vi "Initialization_default.vi"(8 "error in (no error)":errorcluster, 11 "Device Item Ref in":T3 format="%.0x") -> (0 "error out":errorcluster, 3 "Device Item Ref out":T3 format="%.0x")   [LabVIEW 2017, in "ALMA_10201-10401_O2SensorSim System Explorer.lvlib"]
uses:
  ALMA_10201-10401_O2SensorSim System Explorer.lvlib
  <vilib>/NI Veristand/Custom Device API/Custom Device Item Ref.ctl
  Engine/Par.ctl
  Engine/LambdaType.ctl
  <vilib>/NI Veristand/Custom Device API/Set Item Property (String).vi
  <vilib>/NI Veristand/Custom Device API/Custom Device API.lvlib
panel:
  in  "par":T1={"Loop time"={"Period [ms]"=0, "Processor"=0}, "COM"={"COM IP"="0.0.0.0", "COM port"=1, "Local port"=0, "Next_IP 1"=0, "Next_IP 2"=0, "Next_IP 3"=0, "Next_IP 4"=0}, "O2Sensor1"={"Lambda"={"LSU4.2 Lambda"=[], "LSU4.2 Ip"=[], "LSU4.9 Lambda"=[], "LSU4.9 Ip"=[], "LZA03 Lambda"=[], "LZA03 Ip"=[], "LZA08 Lambda"=[], "LZA08 Ip"=[], "Custom Lambda"=[], "Custom Ip"=[]}, "Temp"={"LSU4.2 Temp"=[], "LSU4.2 Ohm"=[], "LSU4.9 Temp"=[], "LSU4.9 Ohm"=[], "LZA03 Temp"=[], "LZA03 Ohm"=[], "LZA08 Temp"=[], "LZA08 Ohm"=[], "Custom Temp"=[], "Custom Ohm"=[]}, "Lambda Type"=0, "PID"={"Ki"=0.0, "Kp"=0.0, "Kd"=0.0, "FeedFW"=0.0}}, "O2Sensor2"={"Lambda"={"LSU4.2 Lambda"=[], "LSU4.2 Ip"=[], "LSU4.9 Lambda"=[], "LSU4.9 Ip"=[], "LZA03 Lambda"=[], "LZA03 Ip"=[], "LZA08 Lambda"=[], "LZA08 Ip"=[], "Custom Lambda"=[], "Custom Ip"=[]}, "Temp"={"LSU4.2 Temp"=[], "LSU4.2 Ohm"=[], "LSU4.9 Temp"=[], "LSU4.9 Ohm"=[], "LZA03 Temp"=[], "LZA03 Ohm"=[], "LZA08 Temp"=[], "LZA08 Ohm"=[], "Custom Temp"=[], "Custom Ohm"=[]}, "Lambda Type"=0, "PID"={"Ki"=0.0, "Kp"=0.0, "Kd"=0.0, "FeedFW"=0.0}}, "O2Sensor3"={"Lambda"={"LSU4.2 Lambda"=[], "LSU4.2 Ip"=[], "LSU4.9 Lambda"=[], "LSU4.9 Ip"=[], "LZA03 Lambda"=[], "LZA03 Ip"=[], "LZA08 Lambda"=[], "LZA08 Ip"=[], "Custom Lambda"=[], "Custom Ip"=[]}, "Temp"={"LSU4.2 Temp"=[], "LSU4.2 Ohm"=[], "LSU4.9 Temp"=[], "LSU4.9 Ohm"=[], "LZA03 Temp"=[], "LZA03 Ohm"=[], "LZA08 Temp"=[], "LZA08 Ohm"=[], "Custom Temp"=[], "Custom Ohm"=[]}, "Lambda Type"=0, "PID"={"Ki"=0.0, "Kp"=0.0, "Kd"=0.0, "FeedFW"=0.0}}, "O2Sensor4"={"Lambda"={"LSU4.2 Lambda"=[], "LSU4.2 Ip"=[], "LSU4.9 Lambda"=[], "LSU4.9 Ip"=[], "LZA03 Lambda"=[], "LZA03 Ip"=[], "LZA08 Lambda"=[], "LZA08 Ip"=[], "Custom Lambda"=[], "Custom Ip"=[]}, "Temp"={"LSU4.2 Temp"=[], "LSU4.2 Ohm"=[], "LSU4.9 Temp"=[], "LSU4.9 Ohm"=[], "LZA03 Temp"=[], "LZA03 Ohm"=[], "LZA08 Temp"=[], "LZA08 Ohm"=[], "Custom Temp"=[], "Custom Ohm"=[]}, "Lambda Type"=0, "PID"={"Ki"=0.0, "Kp"=0.0, "Kd"=0.0, "FeedFW"=0.0}}, "Board"=1, "Mode"=enum."SLSC Mode", "vendor.Num"=4141, "product.Num"=0} {"Board" items=["ALMA-10201", "ALMA-10401"]; "O2Sensor4"."Lambda Type" items=["LSU4.2", "LSU4.9", "LZA03", "LZA08", "Custom", "[mA]"]; "O2Sensor3"."Lambda Type" items=["LSU4.2", "LSU4.9", "LZA03", "LZA08", "Custom", "[mA]"]; "O2Sensor2"."Lambda Type" items=["LSU4.2", "LSU4.9", "LZA03", "LZA08", "Custom", "[mA]"]; "O2Sensor1"."Lambda Type" items=["LSU4.2", "LSU4.9", "LZA03", "LZA08", "Custom", "[mA]"]}
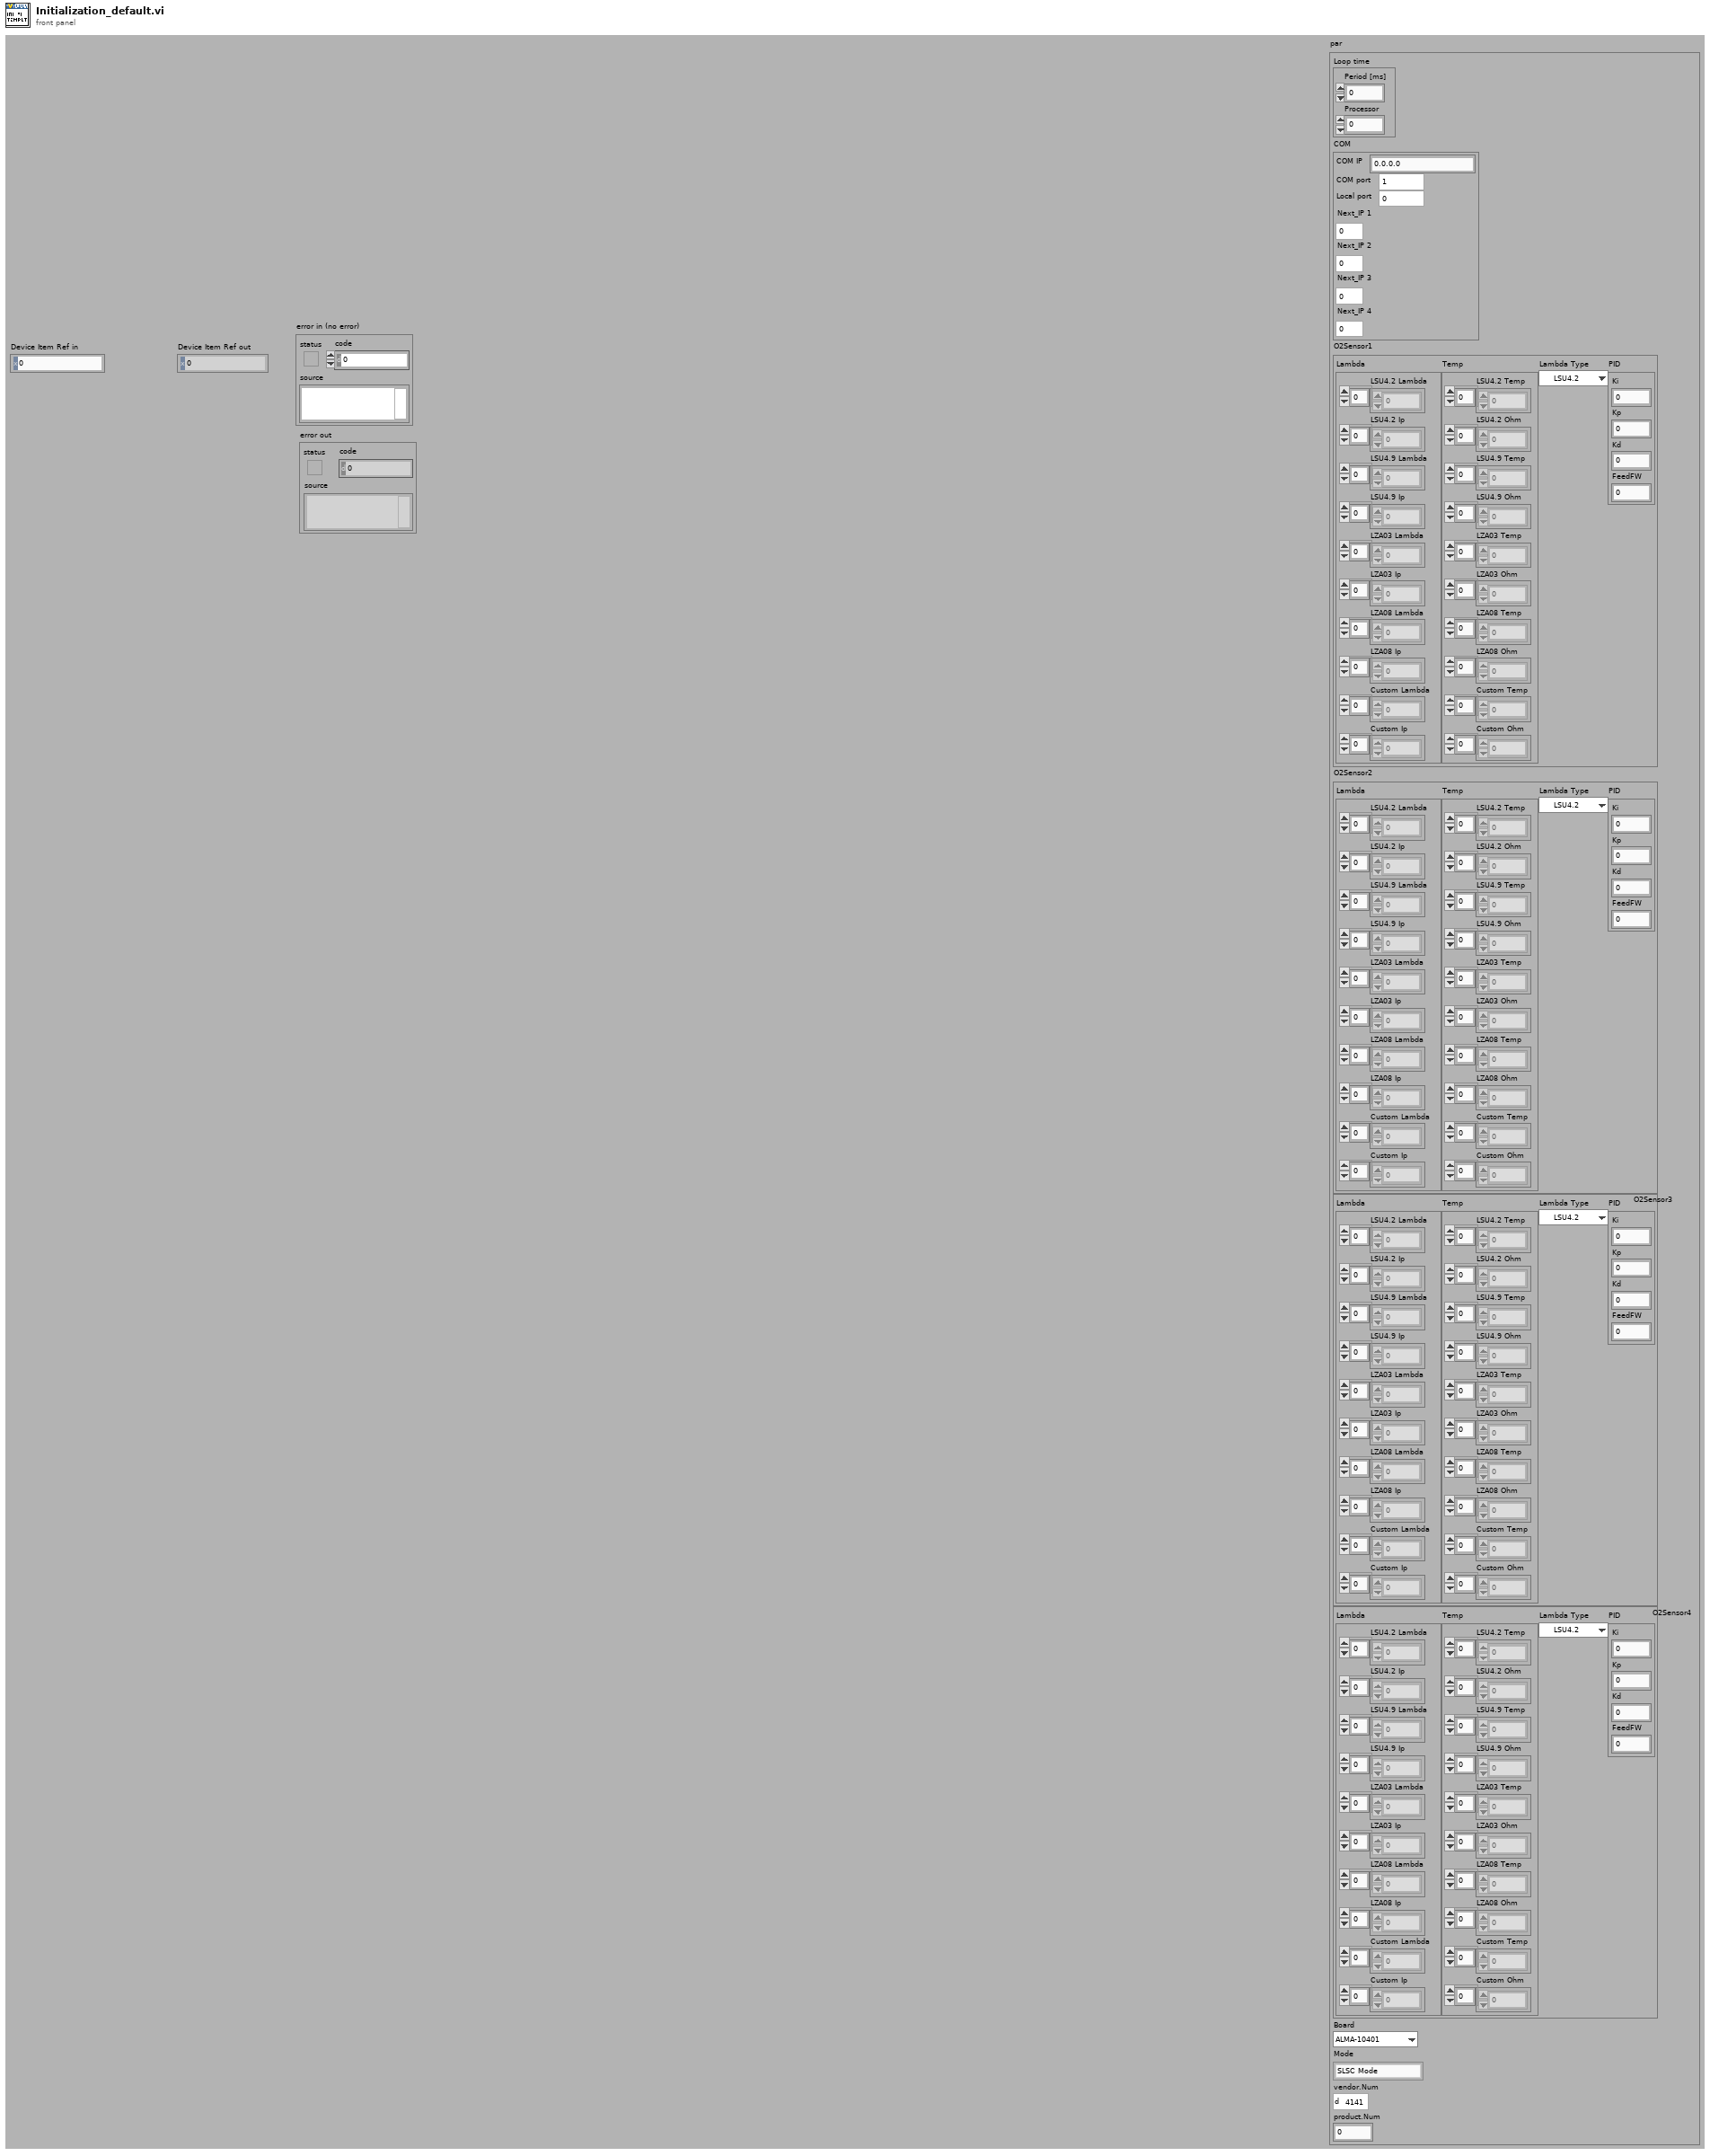
[diagram p1: front panel]
types:
  T1 = typedef "Par.ctl" = cluster{"Loop time":cluster{"Period [ms]":i64, "Processor":i32}, "COM":cluster{"COM IP":string, "COM port":u64, "Local port":u64, "Next_IP 1":u32, "Next_IP 2":u32, "Next_IP 3":u32, "Next_IP 4":u32}, "O2Sensor1":cluster{"Lambda":cluster{"LSU4.2 Lambda":dbl[], "LSU4.2 Ip":dbl[], "LSU4.9 Lambda":dbl[], "LSU4.9 Ip":dbl[], "LZA03 Lambda":dbl[], "LZA03 Ip":dbl[], "LZA08 Lambda":dbl[], "LZA08 Ip":dbl[], "Custom Lambda":dbl[], "Custom Ip":dbl[]}, "Temp":cluster{"LSU4.2 Temp":dbl[], "LSU4.2 Ohm":dbl[], "LSU4.9 Temp":dbl[], "LSU4.9 Ohm":dbl[], "LZA03 Temp":dbl[], "LZA03 Ohm":dbl[], "LZA08 Temp":dbl[], "LZA08 Ohm":dbl[], "Custom Temp":dbl[], "Custom Ohm":dbl[]}, "Lambda Type":T2, "PID":cluster{"Ki":dbl, "Kp":dbl, "Kd":dbl, "FeedFW":dbl}}, "O2Sensor2":cluster{"Lambda":cluster{"LSU4.2 Lambda":dbl[], "LSU4.2 Ip":dbl[], "LSU4.9 Lambda":dbl[], "LSU4.9 Ip":dbl[], "LZA03 Lambda":dbl[], "LZA03 Ip":dbl[], "LZA08 Lambda":dbl[], "LZA08 Ip":dbl[], "Custom Lambda":dbl[], "Custom Ip":dbl[]}, "Temp":cluster{"LSU4.2 Temp":dbl[], "LSU4.2 Ohm":dbl[], "LSU4.9 Temp":dbl[], "LSU4.9 Ohm":dbl[], "LZA03 Temp":dbl[], "LZA03 Ohm":dbl[], "LZA08 Temp":dbl[], "LZA08 Ohm":dbl[], "Custom Temp":dbl[], "Custom Ohm":dbl[]}, "Lambda Type":T2, "PID":cluster{"Ki":dbl, "Kp":dbl, "Kd":dbl, "FeedFW":dbl}}, "O2Sensor3":cluster{"Lambda":cluster{"LSU4.2 Lambda":dbl[], "LSU4.2 Ip":dbl[], "LSU4.9 Lambda":dbl[], "LSU4.9 Ip":dbl[], "LZA03 Lambda":dbl[], "LZA03 Ip":dbl[], "LZA08 Lambda":dbl[], "LZA08 Ip":dbl[], "Custom Lambda":dbl[], "Custom Ip":dbl[]}, "Temp":cluster{"LSU4.2 Temp":dbl[], "LSU4.2 Ohm":dbl[], "LSU4.9 Temp":dbl[], "LSU4.9 Ohm":dbl[], "LZA03 Temp":dbl[], "LZA03 Ohm":dbl[], "LZA08 Temp":dbl[], "LZA08 Ohm":dbl[], "Custom Temp":dbl[], "Custom Ohm":dbl[]}, "Lambda Type":T2, "PID":cluster{"Ki":dbl, "Kp":dbl, "Kd":dbl, "FeedFW":dbl}}, "O2Sensor4":cluster{"Lambda":cluster{"LSU4.2 Lambda":dbl[], "LSU4.2 Ip":dbl[], "LSU4.9 Lambda":dbl[], "LSU4.9 Ip":dbl[], "LZA03 Lambda":dbl[], "LZA03 Ip":dbl[], "LZA08 Lambda":dbl[], "LZA08 Ip":dbl[], "Custom Lambda":dbl[], "Custom Ip":dbl[]}, "Temp":cluster{"LSU4.2 Temp":dbl[], "LSU4.2 Ohm":dbl[], "LSU4.9 Temp":dbl[], "LSU4.9 Ohm":dbl[], "LZA03 Temp":dbl[], "LZA03 Ohm":dbl[], "LZA08 Temp":dbl[], "LZA08 Ohm":dbl[], "Custom Temp":dbl[], "Custom Ohm":dbl[]}, "Lambda Type":T2, "PID":cluster{"Ki":dbl, "Kp":dbl, "Kd":dbl, "FeedFW":dbl}}, "Board":u16, "Mode":enum16{"SLSC Mode", "ANALOG Mode"}, "vendor.Num":u32, "product.Num":u32}
  T2 = typedef "LambdaType.ctl" = u16
  T3 = typedef "Custom Device API.lvlib/Custom Device Item Ref.ctl" = u64
  T4 = cluster{"Lambda":cluster{"LSU4.2 Lambda":dbl[], "LSU4.2 Ip":dbl[], "LSU4.9 Lambda":dbl[], "LSU4.9 Ip":dbl[], "LZA03 Lambda":dbl[], "LZA03 Ip":dbl[], "LZA08 Lambda":dbl[], "LZA08 Ip":dbl[], "Custom Lambda":dbl[], "Custom Ip":dbl[]}, "Temp":cluster{"LSU4.2 Temp":dbl[], "LSU4.2 Ohm":dbl[], "LSU4.9 Temp":dbl[], "LSU4.9 Ohm":dbl[], "LZA03 Temp":dbl[], "LZA03 Ohm":dbl[], "LZA08 Temp":dbl[], "LZA08 Ohm":dbl[], "Custom Temp":dbl[], "Custom Ohm":dbl[]}, "Lambda Type":T2, "PID":cluster{"Ki":dbl, "Kp":dbl, "Kd":dbl, "FeedFW":dbl}}
  T5 = cluster{"Lambda":cluster{"LSU4.2 Lambda":dbl[], "LSU4.2 Ip":dbl[], "LSU4.9 Lambda":dbl[], "LSU4.9 Ip":dbl[], "LZA03 Lambda":dbl[], "LZA03 Ip":dbl[], "LZA08 Lambda":dbl[], "LZA08 Ip":dbl[], "Custom Lambda":dbl[], "Custom Ip":dbl[]}, "Temp":cluster{"LSU4.2 Temp":dbl[], "LSU4.2 Ohm":dbl[], "LSU4.9 Temp":dbl[], "LSU4.9 Ohm":dbl[], "LZA03 Temp":dbl[], "LZA03 Ohm":dbl[], "LZA08 Temp":dbl[], "LZA08 Ohm":dbl[], "Custom Temp":dbl[], "Custom Ohm":dbl[]}, "Lambda Type":T2, "PID":cluster{"Ki":dbl, "Kp":dbl, "Kd":dbl, "FeedFW":dbl}}[]
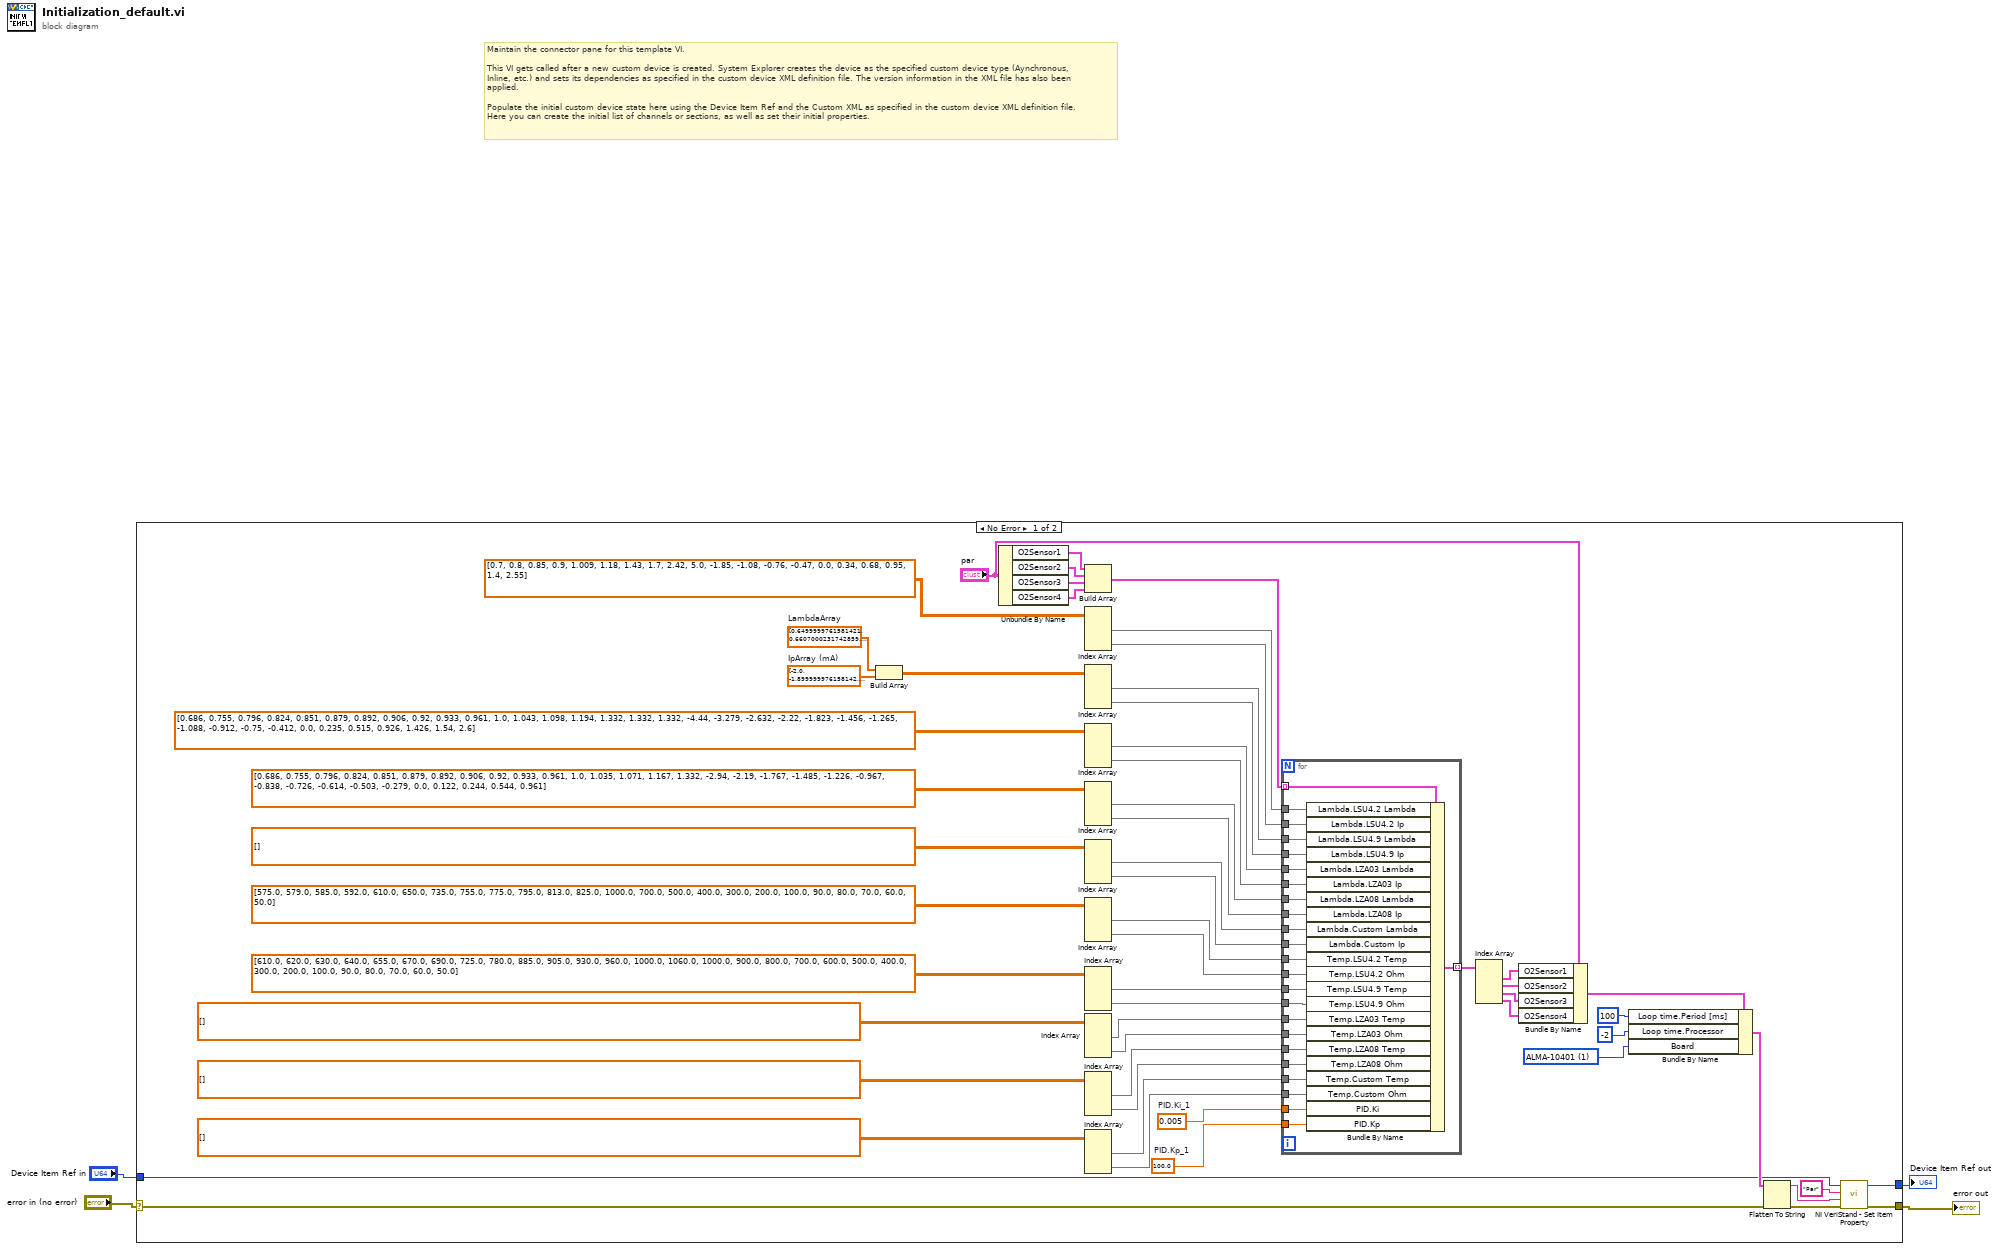
[diagram p0: block diagram]
diagram:
  # "Maintain the connector pane for this template VI.\n\nThis VI gets called after a new custom device is created. System Explorer creates the device as the specified custom device type (Aynchronous, Inline, etc.) and sets its dependencies as specified in the custom device XML definition file. The version information in the XML file has also been applied.\n\nPopulate the initial custom device state here using the Device Item Ref and the Custom XML as specified in the custom device XML definition file. Here you can create the initial list of channels or sections, as well as set their initial properties."
  n1 = case shown="No Error" "error in (no error)" {
    selector: "error in (no error)" -> [w6 w87]
    tunnel: [w60 w87] -> w2
    tunnel: [w61 w86] -> w3
    tunnel: "Device Item Ref in" -> [w7 w86]
    frame No Error {
      w5 = u16 1 items=["ALMA-10201", "ALMA-10401"] ("Board 2")
      w12 = 100.0  # PID.Kp_1
      w13 = 0.005  # PID.Ki_1
      w38 = sgl[] [0.65, 0.6607, 0.6732, 0.6866, 0.7, 0.714, 0.7278, 0.7418, 0.75, 0.7716, 0.7876, 0.7999, 0.8224, 0.841, 0.8502, 0.8802, 0.8999, 0.9501, 0.9791, 0.9895, 1.0, 1.0032, 1.01, 1.0301, 1.0498, 1.077, 1.1, 1.1319, 1.179, 1.1921, 1.2243, 1.2581, 1.3002, 1.331, 1.3703, 1.4289, 1.4554, 1.5016, 1.5504, 1.6021, 1.657, 1.701, 1.7774, 1.8437, 1.9145, 1.9904, 2.0719, 2.1597, 2.2545, 2.3571, 2.4687, 2.5904, 2.7236, 2.8701, 3.0321, 3.212, 3.4131, 3.6393, 3.8958, 4.189, 4.5275, 4.9229, 5.3907, 5.9531, 6.6421, 7.5061, 8.6219, 10.1187, 12.2328, 15.99]  # LambdaArray
      w37 = sgl[] [-2.0, -1.9, -1.8, -1.7, -1.602, -1.5, -1.4, -1.3, -1.243, -1.1, -1.0, -0.927, -0.8, -0.7, -0.652, -0.5, -0.405, -0.183, -0.0746, -0.0398, -0.007, 0.0, 0.0146, 0.057, 0.097, 0.15, 0.193, 0.25, 0.329, 0.35, 0.4, 0.45, 0.509, 0.55, 0.6, 0.67, 0.7, 0.75, 0.8, 0.85, 0.9, 0.938, 1.0, 1.05, 1.1, 1.15, 1.2, 1.25, 1.3, 1.35, 1.4, 1.45, 1.5, 1.55, 1.6, 1.65, 1.7, 1.75, 1.8, 1.85, 1.9, 1.95, 2.0, 2.05, 2.1, 2.15, 2.2, 2.25, 2.3, 2.3565]  # IpArray (mA)
      n2 = Build Array(w38, w37) -> (w36:sgl[][])
      n3 = Unbundle By Name("par") -> ("O2Sensor1"=w31:T4, "O2Sensor2"=w32:T4, "O2Sensor3"=w33:T4, "O2Sensor4"=w34:T4)
      n4 = Build Array(w31, w32, w33, w34) -> (w30:T5)
      n5 = Index Array(array=dbl[][] [[0.7, 0.8, 0.85, 0.9, 1.009, 1.18, 1.43, 1.7, 2.42, 5.0], [-1.85, -1.08, -0.76, -0.47, 0.0, 0.34, 0.68, 0.95, 1.4, 2.55]] ("appended array 2")) -> (element #1=w35:dbl[], element #2=w54:dbl[])  [unwired: 4 in]
      n6 = Index Array(array=w36) -> (element #1=w56:sgl[], element #2=w55:sgl[])  [unwired: 4 in]
      n7 = Index Array(array=dbl[][] [[0.686, 0.755, 0.796, 0.824, 0.851, 0.879, 0.892, 0.906, 0.92, 0.933, 0.961, 1.0, 1.043, 1.098, 1.194, 1.332, 1.332, 1.332], [-4.44, -3.279, -2.632, -2.22, -1.823, -1.456, -1.265, -1.088, -0.912, -0.75, -0.412, 0.0, 0.235, 0.515, 0.926, 1.426, 1.54, 2.6]] ("appended array")) -> (element #1=w51:dbl[], element #2=w50:dbl[])  [unwired: 4 in]
      n8 = Index Array(array=dbl[][] [[0.686, 0.755, 0.796, 0.824, 0.851, 0.879, 0.892, 0.906, 0.92, 0.933, 0.961, 1.0, 1.035, 1.071, 1.167, 1.332], [-2.94, -2.19, -1.767, -1.485, -1.226, -0.967, -0.838, -0.726, -0.614, -0.503, -0.279, 0.0, 0.122, 0.244, 0.544, 0.961]] ("appended array")) -> (element #1=w49:dbl[], element #2=w48:dbl[])  [unwired: 4 in]
      n9 = Index Array(array=dbl[][] [] ("appended array")) -> (element #1=w47:dbl[], element #2=w46:dbl[])  [unwired: 4 in]
      n10 = Index Array(array=dbl[][] [[575.0, 579.0, 585.0, 592.0, 610.0, 650.0, 735.0, 755.0, 775.0, 795.0, 813.0, 825.0], [1000.0, 700.0, 500.0, 400.0, 300.0, 200.0, 100.0, 90.0, 80.0, 70.0, 60.0, 50.0]] ("appended array")) -> (element #1=w23:dbl[], element #2=w22:dbl[])  [unwired: 4 in]
      n11 = Index Array(array=dbl[][] [[610.0, 620.0, 630.0, 640.0, 655.0, 670.0, 690.0, 725.0, 780.0, 885.0, 905.0, 930.0, 960.0, 1000.0, 1060.0], [1000.0, 900.0, 800.0, 700.0, 600.0, 500.0, 400.0, 300.0, 200.0, 100.0, 90.0, 80.0, 70.0, 60.0, 50.0]] ("appended array")) -> (element #1=w21:dbl[], element #2=w20:dbl[])  [unwired: 4 in]
      n12 = Index Array(array=dbl[][] [] ("appended array")) -> (element #1=w19:dbl[], element #2=w18:dbl[])  [unwired: 4 in]
      n13 = Index Array(array=dbl[][] [] ("appended array")) -> (element #1=w17:dbl[], element #2=w16:dbl[])  [unwired: 4 in]
      n14 = Index Array(array=dbl[][] [] ("appended array")) -> (element #1=w15:dbl[], element #2=w14:dbl[])  [unwired: 4 in]
      n15 = for {
        tunnel: w56 -> [w85]
        tunnel: w55 -> [w84]
        tunnel: w54 -> [w83]
        tunnel: w51 -> [w82]
        tunnel: w50 -> [w81]
        tunnel: w49 -> [w80]
        tunnel: w48 -> [w79]
        tunnel: w47 -> [w78]
        tunnel: w46 -> [w77]
        tunnel: w35 -> [w76]
        tunnel: w30 -> [w75] mode=indexing
        tunnel: [w74] -> w25 mode=indexing
        tunnel: w23 -> [w73]
        tunnel: w22 -> [w72]
        tunnel: w21 -> [w71]
        tunnel: w20 -> [w70]
        tunnel: w19 -> [w69]
        tunnel: w18 -> [w68]
        tunnel: w17 -> [w67]
        tunnel: w16 -> [w66]
        tunnel: w15 -> [w65]
        tunnel: w14 -> [w64]
        tunnel: w13 -> [w63]
        tunnel: w12 -> [w62]
        n16 = Bundle By Name(cluster=w75, "Lambda.LSU4.2 Lambda"=w76, "Lambda.LSU4.2 Ip"=w83, "Lambda.LSU4.9 Lambda"=w85, "Lambda.LSU4.9 Ip"=w84, "Lambda.LZA03 Lambda"=w82, "Lambda.LZA03 Ip"=w81, "Lambda.LZA08 Lambda"=w80, "Lambda.LZA08 Ip"=w79, "Lambda.Custom Lambda"=w78, "Lambda.Custom Ip"=w77, "Temp.LSU4.2 Temp"=w73, "Temp.LSU4.2 Ohm"=w72, "Temp.LSU4.9 Temp"=w71, "Temp.LSU4.9 Ohm"=w70, "Temp.LZA03 Temp"=w69, "Temp.LZA03 Ohm"=w68, "Temp.LZA08 Temp"=w67, "Temp.LZA08 Ohm"=w66, "Temp.Custom Temp"=w65, "Temp.Custom Ohm"=w64, "PID.Ki"=w63, "PID.Kp"=w62) -> (w74:T4)
      }
      n17 = Index Array(array=w25) -> (element #1=w26:T4, element #2=w27:T4, element #3=w28:T4, element #4=w29:T4)  [unwired: 4 in]
      n18 = Bundle By Name(cluster="par", "O2Sensor1"=w26, "O2Sensor2"=w27, "O2Sensor3"=w28, "O2Sensor4"=w29) -> (w11:T1)
      n19 = Bundle By Name(cluster=w11, "Loop time.Period [ms]"=i64 100, "Loop time.Processor"=-2, "Board"=w5) -> (w8:T1)
      n20 = Flatten To String(anything=w8, error in (no error)=w6) -> (data string=w57:string, error out=w58:errorcluster)  [unwired: 2 in, 1 out]
      n21 = call-poly <vilib>:"NI VeriStand - Set Item Property.vi"("error in (no error)"=w58, "Value"=w57, "Property Name"="Par", "Item Ref in"=w7) -> ("error out"=w60:errorcluster, "Item Ref out"=w61:T3)  [unwired: 5 in, 1 out]
    }
    frame Error {
    }
  }
  "error out" <- w2
  "Device Item Ref out" <- w3
